vi "CompTrigStartProps.vi"(0 "task in":refnum<k24>, 5 "error in (no error)":errorcluster) -> (7 "AnalogHWTrigSense":i32, 8 "TrigChannelStr":string, 9 "AnalogSWTrigSense":i32, 10 "TriggerChannel":i32, 11 "CounterChanTrigSense":i32, 12 "Variance":dbl, 13 "DigitalPatternTrigSense":i32, 14 "task out":refnum<k24>, 15 "Level":dbl, 16 "Type":i32, 17 "PretriggerCount":i32, 18 "ExtTTLTrigSense":i32, 19 "error out":errorcluster)   [LabVIEW 2010]
uses:
  C:/Program Files/National Instruments/LabVIEW 2010/vi.lib/ULx/ULx_LV.dll
  Program Files/National Instruments/LabVIEW 2010/vi.lib/ULx/ULx_LV.dll
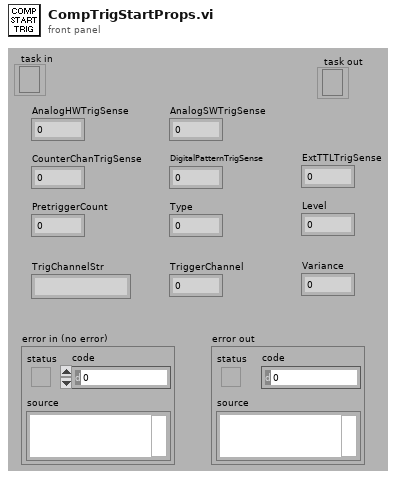
[diagram p1: front panel]
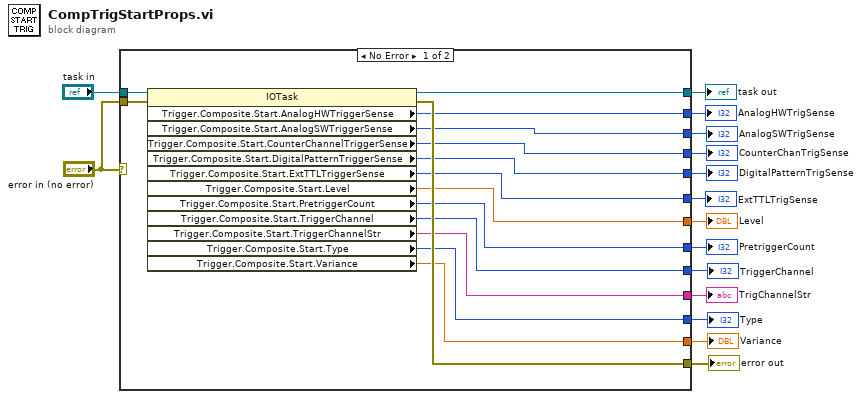
[diagram p0: block diagram]
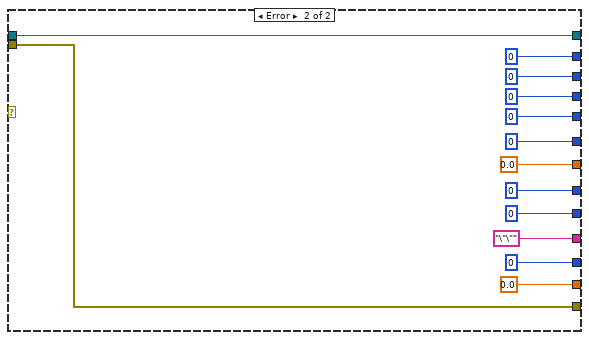
[diagram p2: hidden frame]
diagram:
  n1 = case shown="No Error" "error in (no error)" {
    tunnel: "task in" -> [w30 w43]
    tunnel: "error in (no error)" -> [w28 w42]
    tunnel: [w29 w43] -> w13
    tunnel: [w27 w42] -> w12
    tunnel: [w26 0 ("Trigger.Composite.Start.AnalogHWTriggerSense")] -> w11
    tunnel: [w22 0 ("Trigger.Basic.Type")] -> w10
    tunnel: [w25 0 ("Trigger.Composite.Start.CounterChannelTriggerSense")] -> w9
    tunnel: [w24 0 ("Trigger.Composite.Start.DigitalPatternTriggerSense")] -> w8
    tunnel: [w21 0 ("Trigger.Basic.PretriggerCount")] -> w7
    tunnel: [w20 0.0 ("Trigger.Gated.LowThreshold")] -> w6
    tunnel: [w19 0 ("Trigger.Basic.Slope")] -> w5
    tunnel: [w18 0 ("Trigger.Gated.Type")] -> w4
    tunnel: [w23 "\"\"" ("Trigger.Composite.Start.TriggerChannelStr")] -> w3
    tunnel: [w17 0 ("Trigger.Gated.When")] -> w2
    tunnel: [w16 0.0 ("Trigger.Gated.WindowBottom")] -> w1
    frame No Error {
      n2 = property class="IOTask"(reference=w30, error in=w28) -> (reference out=w29:refnum<k24>, error out=w27:errorcluster, "Trigger.Composite.Start.AnalogHWTriggerSense"=w26:i32, "Trigger.Composite.Start.AnalogSWTriggerSense"=w22:i32, "Trigger.Composite.Start.CounterChannelTriggerSense"=w25:i32, "Trigger.Composite.Start.DigitalPatternTriggerSense"=w24:i32, "Trigger.Composite.Start.ExtTTLTriggerSense"=w21:i32, "Trigger.Composite.Start.Level"=w20:dbl, "Trigger.Composite.Start.PretriggerCount"=w19:i32, "Trigger.Composite.Start.TriggerChannel"=w18:i32, "Trigger.Composite.Start.TriggerChannelStr"=w23:string, "Trigger.Composite.Start.Type"=w17:i32, "Trigger.Composite.Start.Variance"=w16:dbl)
    }
    frame Error {
    }
  }
  "task out" <- w13
  "error out" <- w12
  "AnalogHWTrigSense" <- w11
  "AnalogSWTrigSense" <- w10
  "CounterChanTrigSense" <- w9
  "DigitalPatternTrigSense" <- w8
  "ExtTTLTrigSense" <- w7
  "Level" <- w6
  "PretriggerCount" <- w5
  "TriggerChannel" <- w4
  "TrigChannelStr" <- w3
  "Type" <- w2
  "Variance" <- w1
